vi "Axis Aligned Bounding Box.vi"(10 "Texture Size":refnum<class "Vector 2D.lvclass">, 11 "Element in":refnum<class "Element.lvclass">) -> (3 "AABB":T1)   [LabVIEW 2021, in "Element.lvclass"]
uses:
  Element.lvclass
  Re-use Libraries/Vector 2D/Vector 2D.lvclass
  Element.lvclass/Element.ctl
  Motion/Motion.lvclass/Motion.ctl
  Re-use Libraries/Vector 2D/Vector 2D.lvclass/Vector 2D.ctl
  Motion/Motion.lvclass
  Re-use Libraries/Utility/Typedef/Axis Aligned Bounding Box.ctl
  Re-use Libraries/Utility/Utility.lvlib
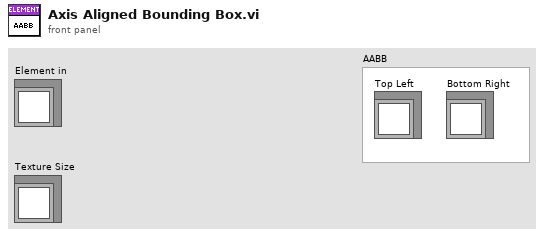
[diagram p1: front panel]
types:
  T1 = typedef "Utility.lvlib/Axis Aligned Bounding Box.ctl" = cluster{"Top Left":refnum<class "Vector 2D.lvclass">, "Bottom Right":refnum<class "Vector 2D.lvclass">}
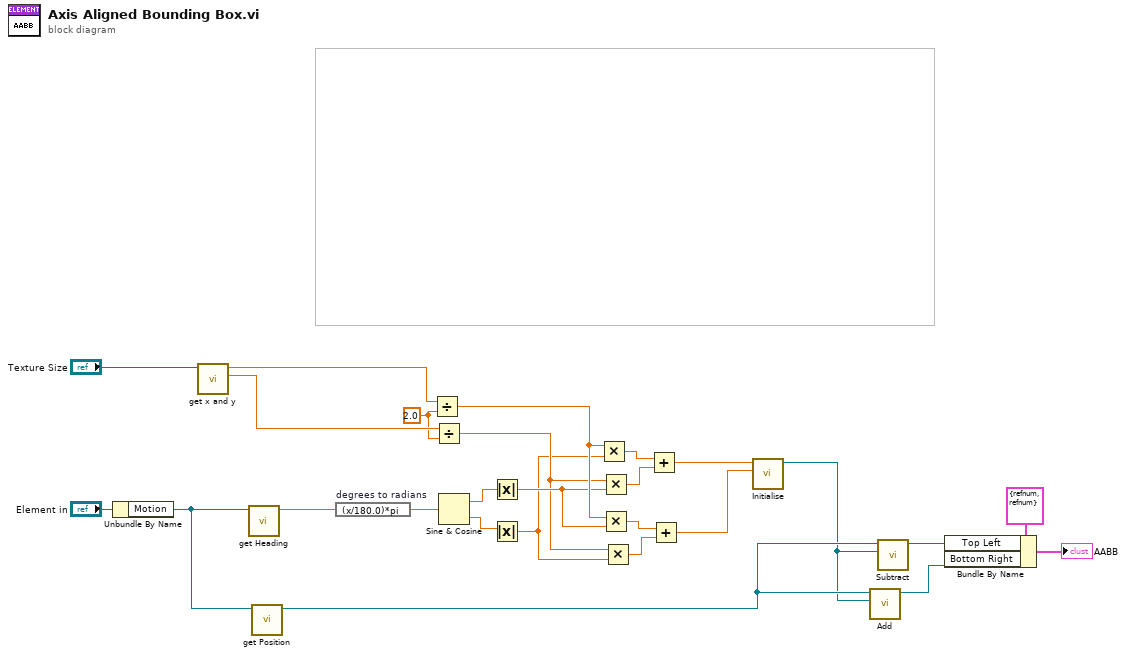
[diagram p0: block diagram]
diagram:
  w17 = sgl 2.0 ("y")
  n1 = Unbundle By Name("Element in") -> ("Motion"=w25:refnum<class "Motion.lvclass">)
  n2 = call "get x and y.vi"("Vector 2D in"="Texture Size") -> ("y"=w18:sgl, "x"=w19:sgl)  [unwired: 9 in]
  n3 = call "get Heading.vi"("Motion in"=w25) -> ("Heading [deg]"=w23:sgl)  [unwired: 10 in]
  n4 = call "get Position.vi"("Motion in"=w25) -> ("Displacement"=w3:refnum<class "Vector 2D.lvclass">)  [unwired: 10 in]
  n5 = expression code="(x/180.0)*pi" "degrees to radians"(w23) -> (w24:sgl)
  n6 = Divide(x=w19, y=w17) -> (x/y=w12:sgl)
  n7 = Divide(x=w18, y=w17) -> (x/y=w10:sgl)
  n8 = Sine & Cosine(0:w24) -> (1:w22:sgl, 2:w21:sgl)
  n9 = Absolute Value(x=w22) -> (abs(x)=w11:sgl)
  n10 = Absolute Value(x=w21) -> (abs(x)=w9:sgl)
  n11 = Multiply(x=w12, y=w9) -> (x*y=w16:sgl)
  n12 = Multiply(x=w10, y=w11) -> (x*y=w15:sgl)
  n13 = Multiply(x=w12, y=w11) -> (x*y=w13:sgl)
  n14 = Multiply(x=w10, y=w9) -> (x*y=w14:sgl)
  n15 = Add(x=w16, y=w15) -> (x+y=w6:sgl)
  n16 = Add(x=w13, y=w14) -> (x+y=w5:sgl)
  n17 = call "Initialise.vi"("y"=w5, "x"=w6) -> ("Vector 2D out"=w2:refnum<class "Vector 2D.lvclass">)  [unwired: 9 in]
  n18 = call "Add.vi"("B"=w2, "A"=w3) -> ("A+B"=w1:refnum<class "Vector 2D.lvclass">)  [unwired: 9 in]
  n19 = call "Subtract.vi"("B"=w2, "A"=w3) -> ("A-B"=w4:refnum<class "Vector 2D.lvclass">)  [unwired: 9 in]
  n20 = Bundle By Name(cluster=T1 {"Top Left"=refnum, "Bottom Right"=refnum} ("AABB"), "Top Left"=w4, "Bottom Right"=w1) -> (→"AABB":T1)
